vi "handleEvtDetails.vi"(8 "error in (no error)":errorcluster, 10 "evtDetails":string, 11 "TcpServer.lvclass":refnum<class "TcpServer.lvclass">) -> (0 "error out":errorcluster, 2 "evtDetailsString":string, 3 "TcpServer.lvclass":refnum<class "TcpServer.lvclass">)   [LabVIEW 2018, in "TcpServer.lvclass"]
uses:
  TcpServer.lvclass
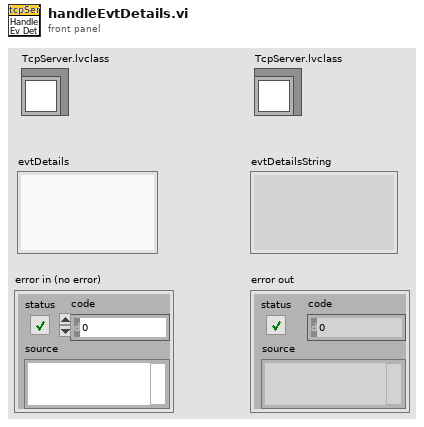
[diagram p1: front panel]
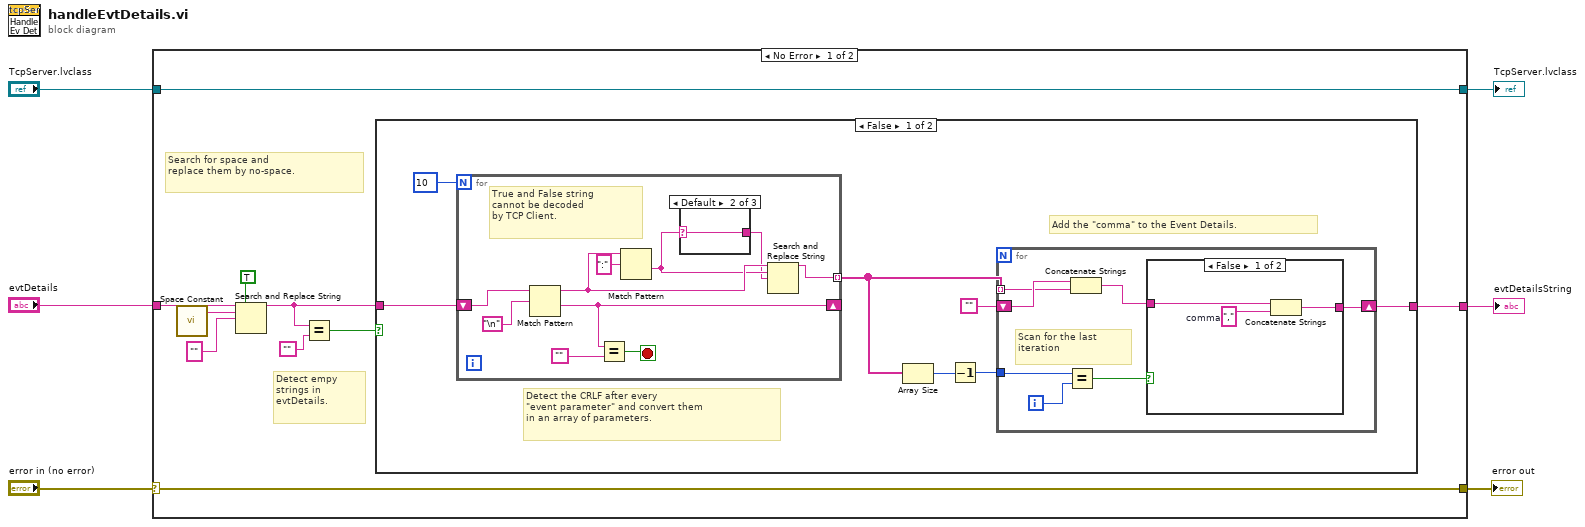
[diagram p0: block diagram]
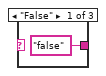
[diagram p3: hidden frame]
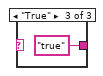
[diagram p4: hidden frame]
diagram:
  n1 = case shown="No Error" "error in (no error)" {
    selector: "error in (no error)" -> [w7 w49]
    tunnel: [w16 _] -> w6
    tunnel: "evtDetails" -> [w12 _]
    tunnel: [w7 w49] -> w3
    tunnel: "TcpServer.lvclass" -> [w15 w50]
    tunnel: [w15 w50] -> w1
    frame No Error {
      # "Search for space and\nreplace them by no-space."
      # "Detect empy\nstrings in \nevtDetails."
      n2 = call <vilib>:"Space Constant.vi"() -> ("String"=w11:string)
      n3 = Search and Replace String(replace all?=TRUE ("replace all? (F)"), input string=w12, search string=w11, replace string="" ("replace string (\"\")")) -> (result string=w9:string)  [unwired: 4 in, 3 out]
      n4 = Equal?(x=w9, y="") -> (x = y?=w13:bool)
      n5 = case shown="False" w13 {
        tunnel: [w23 w48] -> w16
        tunnel: w9 -> [w17 w48]
        frame False {
          # "Add the \"comma\" to the Event Details."
          # "Detect the CRLF after every\n\"event parameter\" and convert them\nin an array of parameters."
          n6 = for {
            N: 10 -> [_]
            tunnel: [w37] -> w20 mode=indexing
            shift-right: [w41] -> _
            shift-left: w17 -> [w43]
            stop <- w42 stop-if-true
            # "True and False string\ncannot be decoded\nby TCP Client."
            n7 = Match Pattern(string=w43, regular expression="\n") -> (before substring=w38:string, after substring=w41:string)  [unwired: 1 in, 2 out]
            n8 = Equal?(x=w41, y="") -> (x = y?=w42:bool)
            n9 = Match Pattern(string=w38, regular expression=":") -> (after substring=w36:string)  [unwired: 1 in, 3 out]
            n10 = case shown="Default" w36 {
              selector: w36 -> [_ w46 _]
              tunnel: ["false" ("regular expression") w46 "true" ("regular expression")] -> w35
              frame "False" {
              }
              frame Default {
              }
              frame "True" {
              }
            }
            n11 = Search and Replace String(input string=w38, search string=w36, replace string=w35) -> (result string=w37:string)  [unwired: 5 in, 3 out]
          }
          n12 = Array Size(array=w20) -> (size(s)=w21:i32)
          n13 = Decrement(x=w21) -> (x-1=w22:i32)
          n14 = for {
            tunnel: w20 -> [w29] mode=indexing
            shift-right: [w27] -> w23
            shift-left: "" -> [w30]
            tunnel: w22 -> [w25]
            i -> [w26]
            # "Scan for the last\niteration"
            n15 = Equal?(x=w25, y=w26) -> (x = y?=w24:bool)
            n16 = Concatenate Strings(w30, w29) -> (w28:string)
            n17 = case shown="False" w24 {
              tunnel: w28 -> [w33 w34]
              tunnel: [w32 w34] -> w27
              frame False {
                w31 = ","  # comma
                n18 = Concatenate Strings(w33, w31) -> (w32:string)
              }
              frame True {
                # "In last iteration we\ndon´t add the \\r\\n"
              }
            }
          }
        }
        frame True {
        }
      }
    }
    frame Error {
    }
  }
  "evtDetailsString" <- w6
  "error out" <- w3
  "TcpServer.lvclass" <- w1
